vi "sys_append_symbols.vi"(11 "raw symbols":cdb[](array[numeric])) -> (3 "appended symbols":cdb[](array[numeric]))   [LabVIEW 2014]
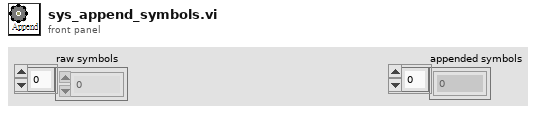
[diagram p1: front panel]
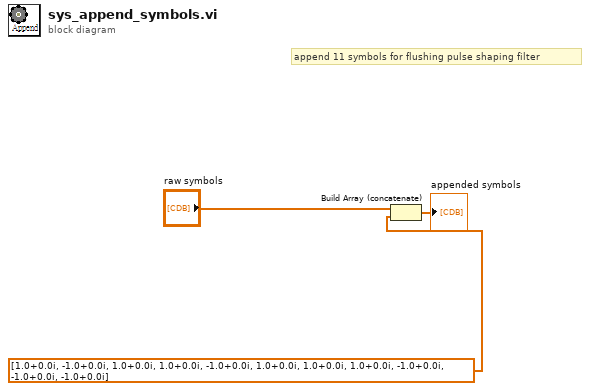
[diagram p0: block diagram]
diagram:
  # "append 11 symbols for flushing pulse shaping filter"
  n1 = Build Array (concatenate)("raw symbols", cdb[] [1.0+0.0i, -1.0+0.0i, 1.0+0.0i, 1.0+0.0i, -1.0+0.0i, 1.0+0.0i, 1.0+0.0i, 1.0+0.0i, -1.0+0.0i, -1.0+0.0i, -1.0+0.0i]) -> (→"appended symbols":cdb[])
